vi "execute.vi"(8 "error in (no error)":errorcluster, 9 "image assembler in":refnum<class "GenericComponent.lvclass">, 10 "imaging mode in":refnum<class "GenericComponent.lvclass">, 11 "DL090309ImagingModeToImageAssemblerAdapter in":refnum<class "AdapterDL090309ImagingModeToImageAssembler.lvclass">) -> (0 "error out":errorcluster, 1 "image assembler out":refnum<class "GenericComponent.lvclass">, 2 "imaging mode out":refnum<class "GenericComponent.lvclass">, 3 "DL090309ImagingModeToImageAssemblerAdapter out":refnum<class "AdapterDL090309ImagingModeToImageAssembler.lvclass">)   [LabVIEW 2010, in "AdapterDL090309ImagingModeToImageAssembler.lvclass"]
uses:
  AdapterDL090309ImagingModeToImageAssembler.lvclass
  common/classes/GenericComponent/GenericComponent/GenericComponent.lvclass
  ImageAssembler/ImageAssemblerDL090211Frame/ImageAssemblerDL090211Frame/ImageAssemblerDL090211Frame.lvclass
  ImagingMode/ImagingModeDL090130Frame/ImagingModeDL090130Frame/ImagingModeDL090130Frame.lvclass
  ImageAssembler/ImageAssemblerDL090211Scaffold/ImageAssemblerDL090211Scaffold/ImageAssemblerDL090211Scaffold.lvclass
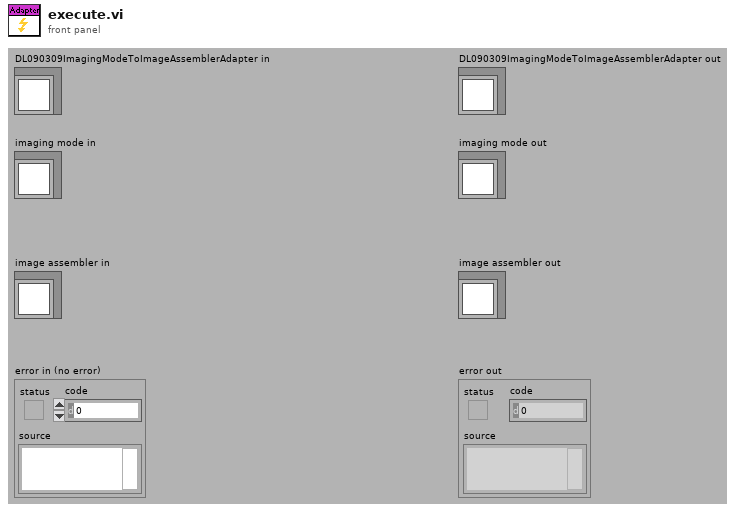
[diagram p1: front panel]
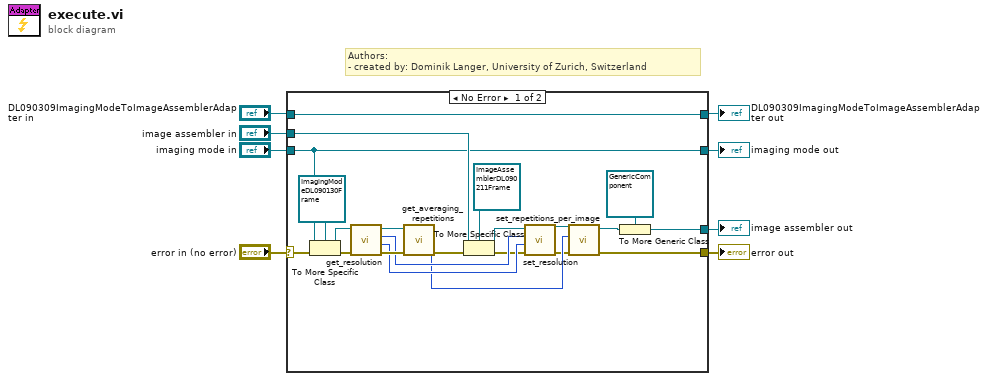
[diagram p0: block diagram]
diagram:
  # "Authors: \n- created by: Dominik Langer, University of Zurich, Switzerland"
  n1 = case shown="No Error" "error in (no error)" {
    selector: "error in (no error)" -> [w16 w34]
    tunnel: [w10 w34] -> w7
    tunnel: [w14 w33] -> w5
    tunnel: "DL090309ImagingModeToImageAssemblerAdapter in" -> [w14 w33]
    tunnel: "imaging mode in" -> [w12 w31]
    tunnel: "image assembler in" -> [w15 w32]
    tunnel: [w13 w32] -> w2
    tunnel: [w12 w31] -> w1
    frame No Error {
      n2 = To More Specific Class(target class=refnum<class "ImagingModeDL090130Frame.lvclass"> refnum ("DL090130FrameScanMode.lvclass"), reference=w12, error in=w16) -> (specific class reference=w25:refnum<class "ImagingModeDL090130Frame.lvclass">, error out=w26:errorcluster)
      n3 = call-dynamic "get_resolution.vi"("error in (no error)"=w26, "ImagingModeDL090130Frame in"=w25) -> ("error out"=w24:errorcluster, "y resolution"=w21:i32, "x resolution"=w22:i32, "ImagingModeDL090130Frame out"=w23:refnum<class "ImagingModeDL090130Frame.lvclass">)  [unwired: 6 out]
      n4 = call-dynamic "get_averaging_repetitions.vi"("error in (no error)"=w24, "ImagingModeDL090130Frame in"=w23) -> ("error out"=w9:errorcluster, "averaging repetitions"=w19:i32)  [unwired: 8 out]
      n5 = To More Specific Class(target class=refnum<class "ImageAssemblerDL090211Frame.lvclass"> refnum ("DL090211FrameImageAssembler.lvclass"), reference=w15, error in=w9) -> (specific class reference=w27:refnum<class "ImageAssemblerDL090211Frame.lvclass">, error out=w20:errorcluster)
      n6 = call "set_resolution.vi"("error in (no error)"=w20, "y resolution"=w21, "x resolution"=w22, "DL090211FrameImageAssembler.lvclass in"=w27) -> ("error out"=w18:errorcluster, "DL090211FrameImageAssembler.lvclass out"=w30:refnum<class "ImageAssemblerDL090211Frame.lvclass">)  [unwired: 6 out]
      n7 = call "set_repetitions_per_image.vi"("error in (no error)"=w18, "repetitions per image"=w19, "DL090211ImageAssemblerScaffold.lvclass in"=w30) -> ("error out"=w10:errorcluster, "DL090211ImageAssemblerScaffold.lvclass out"=w11:refnum<class "ImageAssemblerDL090211Frame.lvclass">)  [unwired: 7 out]
      n8 = To More Generic Class(target class=refnum<class "GenericComponent.lvclass"> refnum ("GenericComponent.lvclass"), reference=w11) -> (generic class reference=w13:refnum<class "GenericComponent.lvclass">)
    }
    frame Error {
    }
  }
  "error out" <- w7
  "DL090309ImagingModeToImageAssemblerAdapter out" <- w5
  "image assembler out" <- w2
  "imaging mode out" <- w1
